vi "Convert Tesla to Oersted.vi"(2 "Field Rate (T/min)":dbl, 3 "Field (T)":dbl) -> (0 "Field Rate (Oe/s)":dbl, 1 "Field (Oe)":dbl)   [LabVIEW 2019, in "instrument.PPMS.lvclass"]
uses:
  instrument.PPMS.lvclass
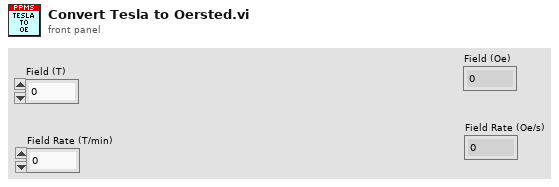
[diagram p1: front panel]
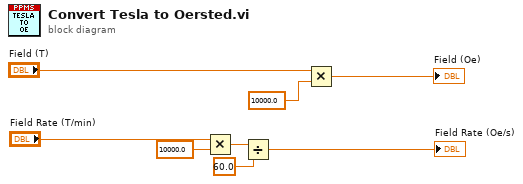
[diagram p0: block diagram]
diagram:
  n1 = Multiply(x="Field Rate (T/min)", y=10000.0) -> (x*y=w2:dbl)
  n2 = Divide(x=w2, y=60.0) -> (x/y=→"Field Rate (Oe/s)":dbl)
  n3 = Multiply(x="Field (T)", y=10000.0) -> (x*y=→"Field (Oe)":dbl)
